vi "proyecto2.vi"() -> ()   [LabVIEW 2012]
panel:
  in  "Frecuenca Alto":dbl=100.0 caption="Lower Cut-Off"
  in  "Tipo de Onda":T1(ring)
  in  "Frecuencia Bajo":dbl=100.0 caption="Lower Cut-Off"
  out "Señal Filtrada":dynamicdata(graph)
  out "Señal Original":waveform(dbl)[](graph)
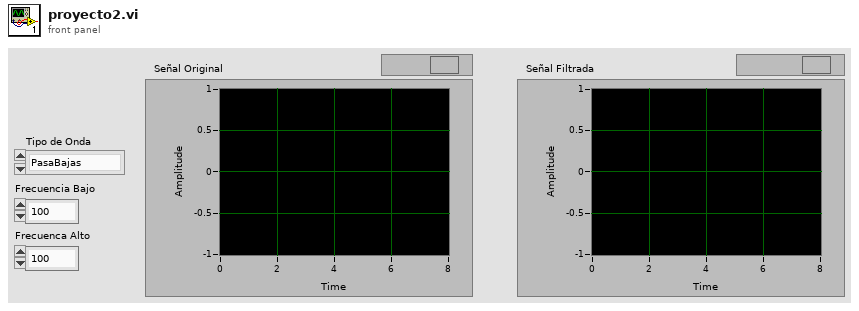
[diagram p1: front panel]
types:
  T1 = enum16{"PasaBajas", "PasaAltas", "PasaBanda", "RechazaBanda"}
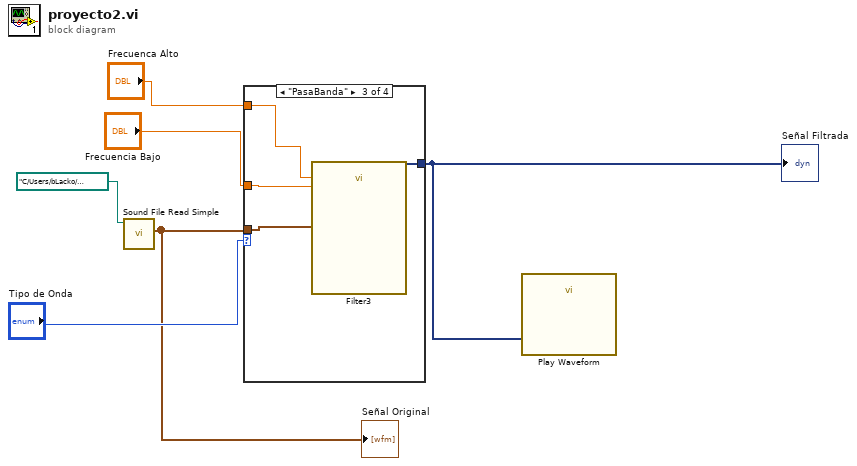
[diagram p0: block diagram]
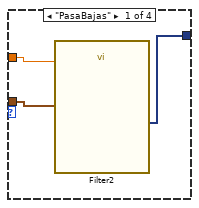
[diagram p2: hidden frame]
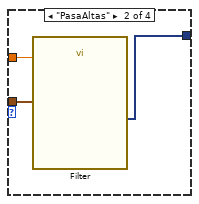
[diagram p3: hidden frame]
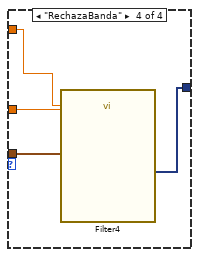
[diagram p4: hidden frame]
diagram:
  n1 = call <vilib>:"Sound File Read Simple.vi"("path"=path "C:/Users/bLacko/Desktop/A todo Unipoli/Transformadas y Series/tonoacdc.wav") -> ("data"=w2:waveform(dbl)[])  [unwired: 7 in, 3 out]
  "Señal Original" <- w2
  n2 = case shown="\"PasaBanda\"" "Tipo de Onda" {
    tunnel: w2 -> [w8 w12 w15 w19]
    tunnel: "Frecuencia Bajo" -> [w9 w11 w16 w20]
    tunnel: [w7 w10 w14 w18] -> w1
    tunnel: "Frecuenca Alto" -> [_ _ w13 w17]
    frame "PasaBajas" {
      n3 = call "Filter2"("Lower Cut-Off"=w9, "Signal"=w8) -> ("Filtered Signal"=w7:dynamicdata)  [unwired: 8 in, 1 out]
    }
    frame "PasaAltas" {
      n4 = call "Filter"("Lower Cut-Off"=w11, "Signal"=w12) -> ("Filtered Signal"=w10:dynamicdata)  [unwired: 8 in, 1 out]
    }
    frame "PasaBanda" {
      n5 = call "Filter3"("Lower Cut-Off"=w16, "Upper Cut-Off"=w13, "Signal"=w15) -> ("Filtered Signal"=w14:dynamicdata)  [unwired: 7 in, 1 out]
    }
    frame "RechazaBanda" {
      n6 = call "Filter4"("Lower Cut-Off"=w20, "Upper Cut-Off"=w17, "Signal"=w19) -> ("Filtered Signal"=w18:dynamicdata)  [unwired: 7 in, 1 out]
    }
  }
  "Señal Filtrada" <- w1
  n7 = call "Play Waveform"("Data"=w1) -> ()  [unwired: 18 in, 1 out]
